vi "Principal.vi"() -> ()   [LabVIEW 2016]
uses:
  Microsoft.Kinect
  numero_imagens.vi
  <vilib>/Utility/file.llb/Write Delimited Spreadsheet (DBL).vi
  Software_TCC/historico_dados.vi
  <vilib>/University of Leeds/Kinesthesia Toolkit for Microsoft Kinect/_Polymorphic Close/Close-Skeleton and Video.vi
  <vilib>/University of Leeds/Kinesthesia Toolkit for Microsoft Kinect/_Polymorphic Configure/Event-Skeleton and Video.vi
  <vilib>/3D Express/3D Express.lvlib
panel:
  out "error out":errorcluster
  out "Status":enum16{"Default", "Aquisitar", "Calibrar Joint"}(ring)
  out "Calibraçã":bool
  in  "Cluster":T1={"Save"=FALSE, "membro"="Anatomia", "membro 2"=" Visualização", "anatomia"="Mão Esquerda", "aquisitar"=FALSE, "limpar"=FALSE, "membro"=FALSE, "calibrar_corpo"=FALSE}
  in  "Sair":bool
  in  "seleção_dados":enum32{"Capturar", "Exportar", "Config"}(tab)
  out "aceleração":dbl[](graph)
  out "velocidade":dbl[](graph)
  out "deslocamento":dbl[](graph)
  in  "kinect":string(combo)="Selecione o Kinect"
  in  "Kinect 1":string(combo)="0"
  in  "RGB":bool
  in  "membro 2":string="Status dos Kinects"
  in  "membro":string="Elevação da Câmera"
  in  "Kinect 1":bool
  out "Kinect":picture
  in  "iniciar_calibração":bool
  out "Calibrando membros":u8(slide) scale=0.0..255.0 scale format="%.6f"
  in  "Menus":enum32{"Radio Selection 4", "Radio Selection 3"}(radio)
  out "3D Picture":refnum<vi>(3d-picture)
  # "Ajustes das câmeras do Kinect"
  # "Aguarge . . ."
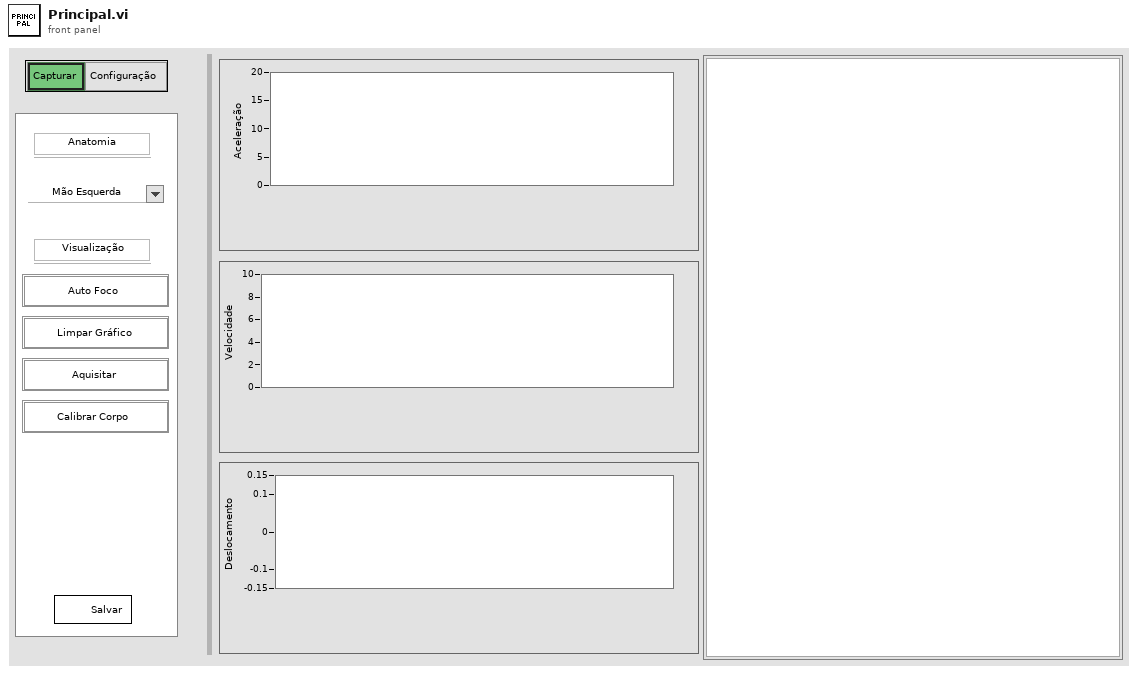
[diagram p1: front panel]
types:
  T1 = cluster{"Save":bool, "membro":string, "membro 2":string, "anatomia":string, "aquisitar":bool, "limpar":bool, "membro":bool, "calibrar_corpo":bool}
  T2 = enum8{"Enabled", "Disabled", "Disabled and Grayed Out"}
  T3 = cluster{"Scene":refnum<vi>, "Joints":refnum<vi>[], "Bones":refnum<vi>[]}
  T4 = cluster{"reference out":refnum<k24>, "KinectSensors":refnum<k24>, "SkeletonStream":refnum<k24>, "ColorStream":refnum<k24>, refnum<k24>[], "get_Item":refnum<k24>}
  T5 = cluster{cluster{"reference out":refnum<k24>, "KinectSensors":refnum<k24>}, "get_Item":refnum<k24>}
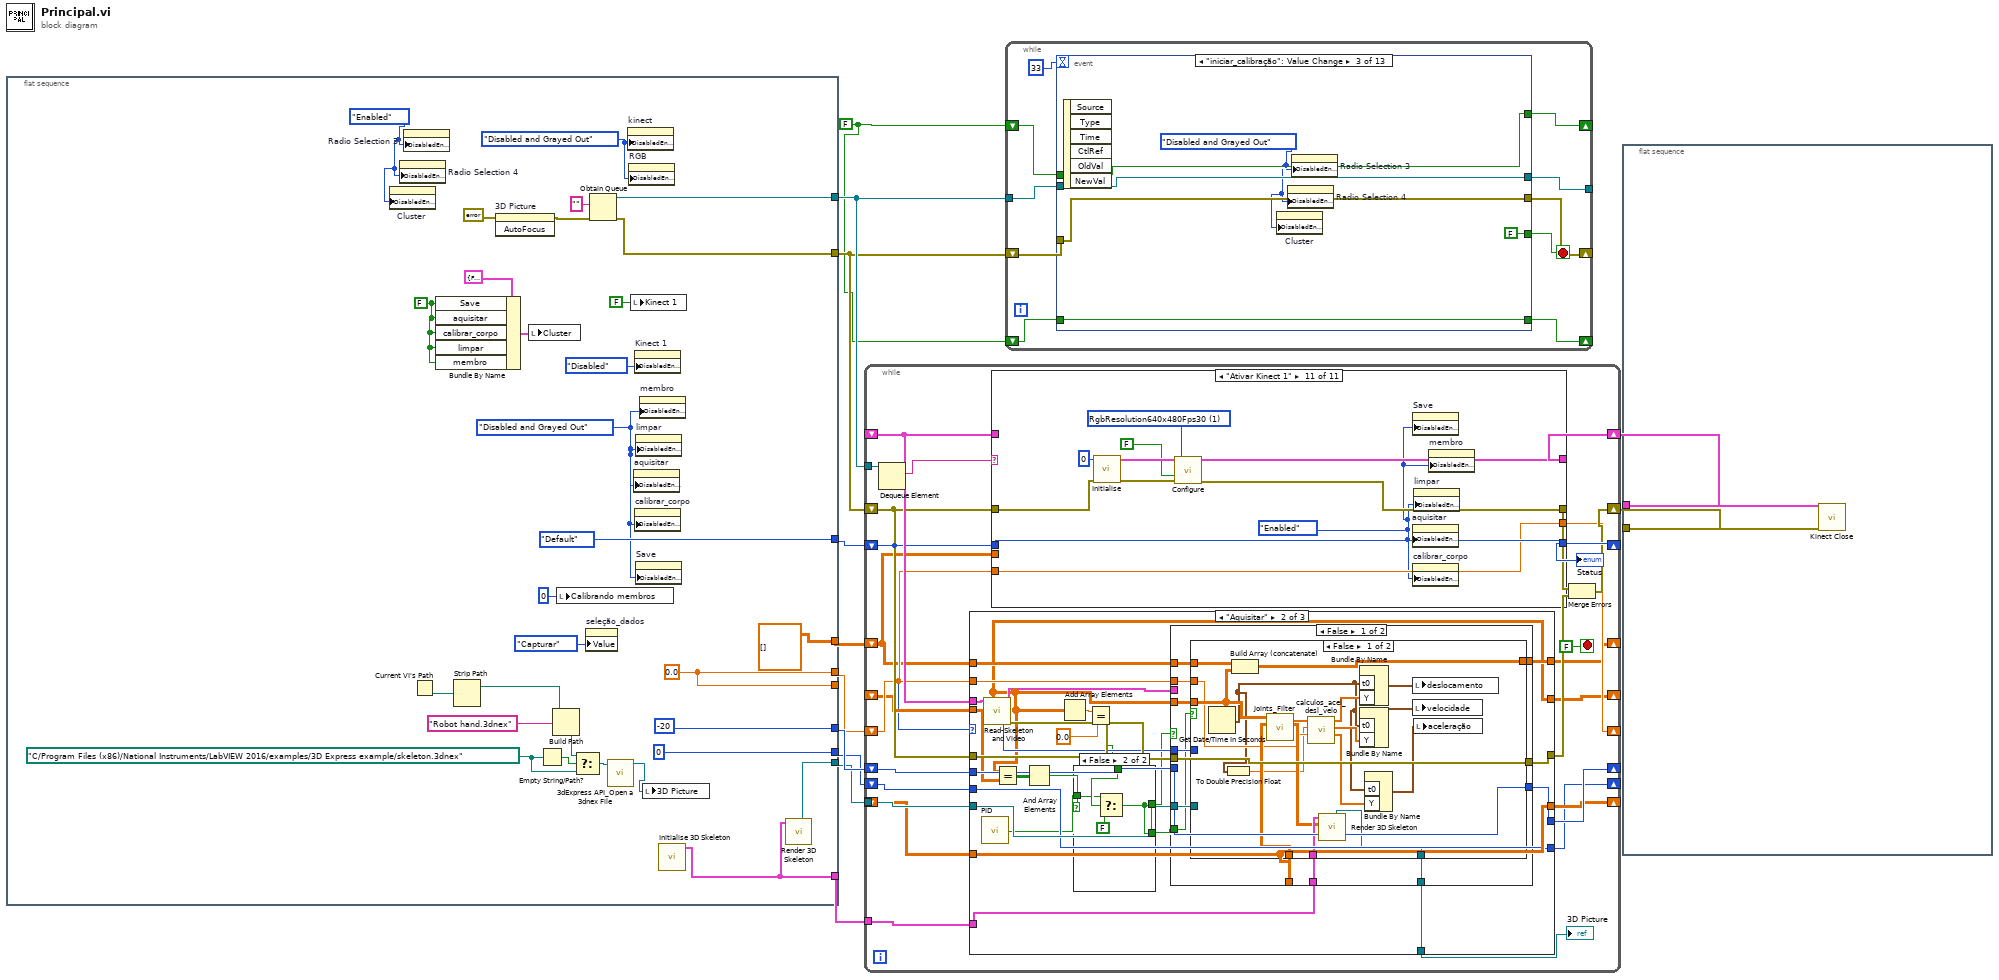
[diagram p0: block diagram]
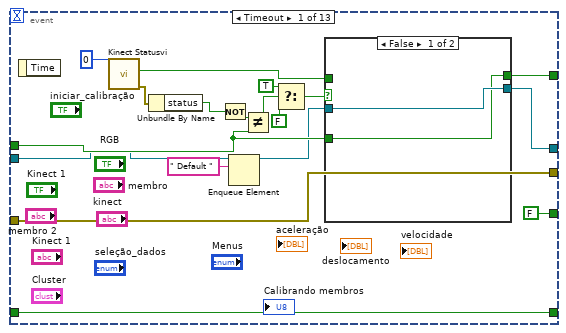
[diagram p2: hidden frame]
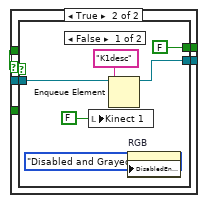
[diagram p3: hidden frame]
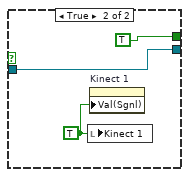
[diagram p4: hidden frame]
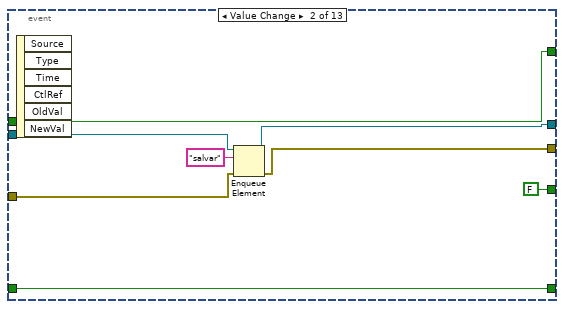
[diagram p5: hidden frame]
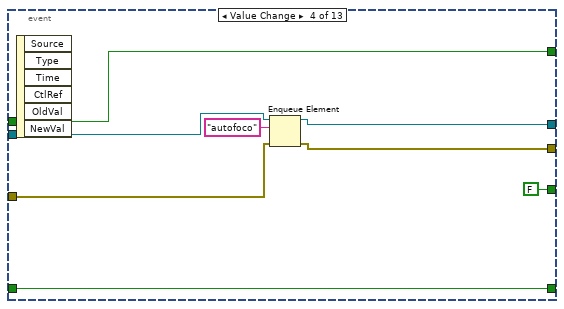
[diagram p6: hidden frame]
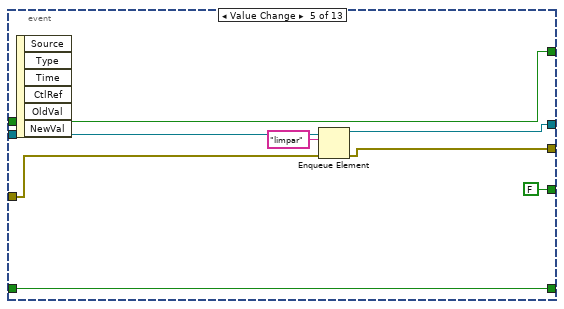
[diagram p7: hidden frame]
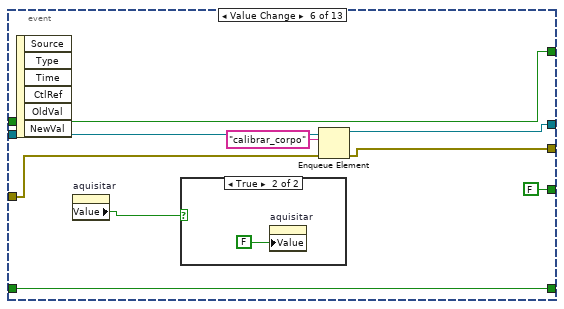
[diagram p8: hidden frame]
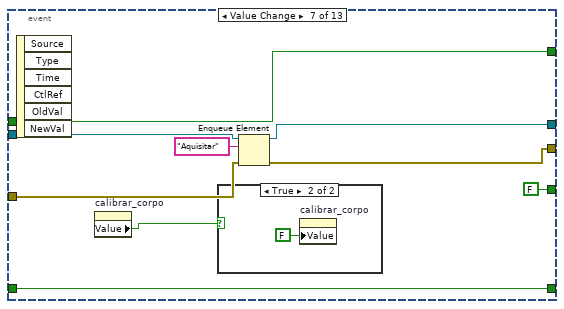
[diagram p10: hidden frame]
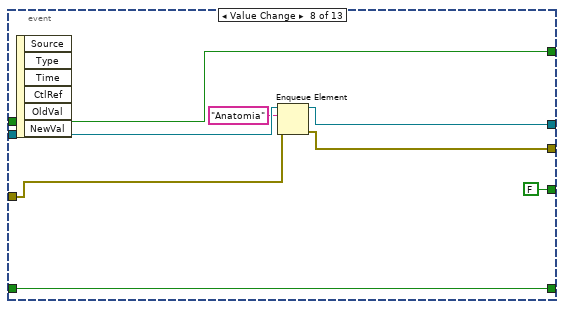
[diagram p12: hidden frame]
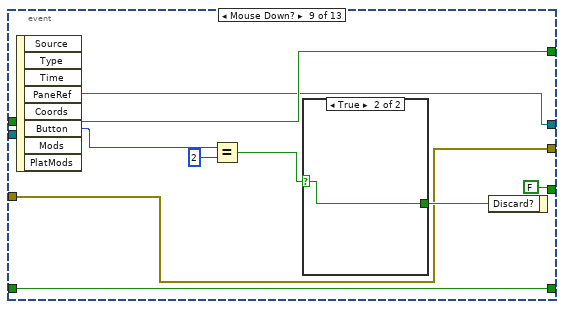
[diagram p13: hidden frame]
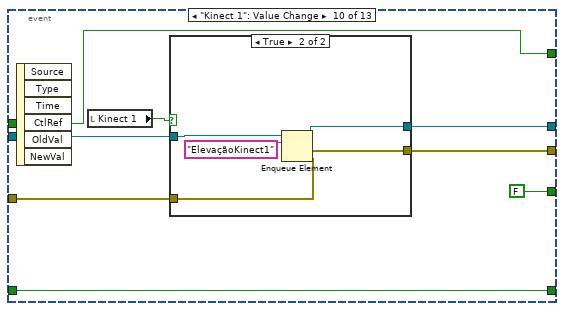
[diagram p15: hidden frame]
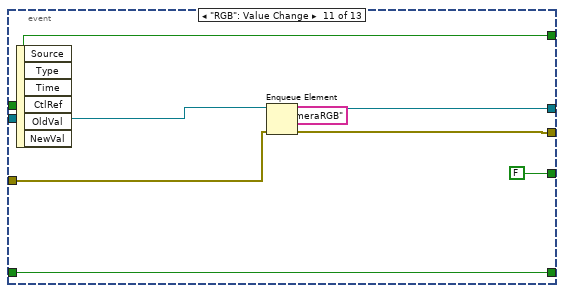
[diagram p17: hidden frame]
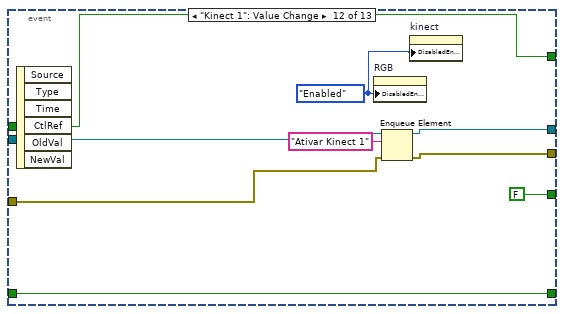
[diagram p18: hidden frame]
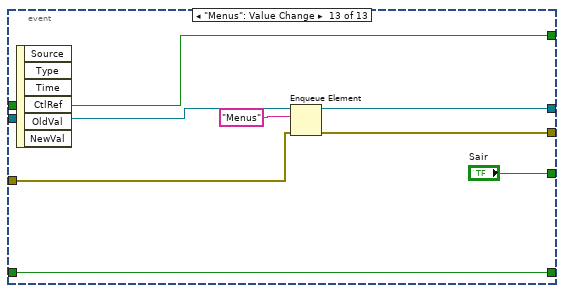
[diagram p19: hidden frame]
diagram:
  w9 = FALSE
  n1 = flat-sequence {
    tunnel: [w41] -> w12
    tunnel: [w40] -> w11
    tunnel: [enum16{"Default", "Aquisitar", "Calibrar Joint"}."Default"] -> w8
    tunnel: [-20] -> w7
    tunnel: [w26] -> w6
    tunnel: [w14] -> w4
    tunnel: [w26] -> _
    tunnel: [0] -> w3
    tunnel: [w16] -> w2
    tunnel: [dbl[][][] []] -> w1
    frame #0 {
      w13 = T2."Enabled" ("Disabled")
      w18 = FALSE ("Save")
      w23 = T2."Disabled and Grayed Out" ("Disabled")
      w28 = path "C:/Program Files (x86)/National Instruments/LabVIEW 2016/examples/3D Express example/skeleton.3dnex" ("File Path Control")
      w26 = 0.0
      w39 = T2."Disabled and Grayed Out" ("Disabled")
      n2 = property on="Cluster" class="Clust (strict)"("DisabledEnum"=w13) -> ()  [unwired: 2 in, 2 out]
      n3 = property on="Radio Selection 4" class="Bool (strict)"("DisabledEnum"=w13) -> ()  [unwired: 2 in, 2 out]
      n4 = property on="Radio Selection 3" class="Bool (strict)"("DisabledEnum"=w13) -> ()  [unwired: 2 in, 2 out]
      n5 = Current VI's Path() -> (path=w31:path)
      n6 = Bundle By Name(cluster=T1 {"Save"=FALSE, "membro"="Anatomia", "membro 2"=" Visualização", "anatomia"="Ombro Esquerdo", "aquisitar"=FALSE, "limpar"=FALSE, "membro"=FALSE, "calibrar_corpo"=FALSE} ("Cluster"), "Save"=w18, "aquisitar"=w18, "calibrar_corpo"=w18, "limpar"=w18, "membro"=w18) -> (w19:T1)
      n7 = Strip Path(path=w31) -> (stripped path=w30:path)  [unwired: 1 out]
      n8 = invoke on="3D Picture" class="SceneGraphDisp (strict)" method="AutoFocus"(error in=errorcluster {"status"=FALSE, "code"=0, "source"=""} ("error constant")) -> (error out=w35:errorcluster)  [unwired: 2 in, 2 out]
      n9 = local write "Cluster"(w19) -> ()
      n10 = Empty String/Path?(string/path=w28) -> (empty?=w29:bool)
      n11 = Build Path(base path=w30, name or relative path="Robot hand.3dnex") -> (appended path=w33:path)
      n12 = local write "Calibrando membros"(u8 0 ("Calibrando membros")) -> ()
      n13 = Select(t=w33, s=w29, f=w28) -> (s? t:f=w34:path)
      n14 = property on="seleção_dados" class="TabCtl (strict)"("Value"=enum32{"Capturar", "Exportar", "Config"}."Capturar" ("seleção_dados")) -> ()  [unwired: 2 in, 2 out]
      n15 = Obtain Queue(element data type="", error in (no error)=w35) -> (queue out=w41:refnum<queue>, error out=w40:errorcluster)  [unwired: 3 in, 1 out]
      n16 = call <vilib>:"3dExpress API_Open a 3dnex File.vi"("selected path"=w34) -> ("Scene out"=w15:refnum<vi>)  [unwired: 8 in, 2 out]
      n17 = property on="kinect" class="CmbBox"("DisabledEnum"=w39) -> ()  [unwired: 2 in, 2 out]
      n18 = property on="RGB" class="Bool"("DisabledEnum"=w39) -> ()  [unwired: 2 in, 2 out]
      n19 = local write "Kinect 1"(FALSE ("Kinect 1")) -> ()
      n20 = property on="aquisitar" class="Bool (strict)"("DisabledEnum"=w23) -> ()  [unwired: 2 in, 2 out]
      n21 = property on="Kinect 1" class="Bool (strict)"("DisabledEnum"=T2."Disabled" ("Disabled")) -> ()  [unwired: 2 in, 2 out]
      n22 = property on="calibrar_corpo" class="Bool (strict)"("DisabledEnum"=w23) -> ()  [unwired: 2 in, 2 out]
      n23 = property on="limpar" class="Bool (strict)"("DisabledEnum"=w23) -> ()  [unwired: 2 in, 2 out]
      n24 = property on="Save" class="Bool (strict)"("DisabledEnum"=w23) -> ()  [unwired: 2 in, 2 out]
      n25 = property on="membro" class="Bool (strict)"("DisabledEnum"=w23) -> ()  [unwired: 2 in, 2 out]
      n26 = local write "3D Picture"(w15) -> ()
      n27 = call <vilib>:"Initialise 3D Skeleton.vi"() -> ("Scene & Skeleton Refs"=w16:T3)  [unwired: 10 in, 1 out]
      n28 = call <vilib>:"Render 3D Skeleton.vi"("Scene & Skeleton Refs In"=w16) -> ("Scene Out"=w14:refnum<vi>)  [unwired: 7 in, 3 out]
    }
  }
  n29 = while {
    tunnel: w12 -> [w67]
    shift-right: [w57] -> w5
    shift-left: w11 -> [w62]
    shift-right: [w65] -> w10
    shift-left: _ -> [w63]
    shift-right: [w64] -> _
    shift-left: w8 -> [w43]
    shift-right: [w60] -> _
    shift-left: w7 -> [w61]
    shift-right: [w56] -> _
    shift-left: w6 -> [w55]
    tunnel: w4 -> [w54]
    shift-right: [w53] -> _
    shift-left: _ -> [w52]
    shift-right: [w51] -> _
    shift-left: _ -> [w49]
    shift-right: [w48] -> _
    shift-left: w3 -> [w50]
    tunnel: w2 -> [w46]
    shift-right: [w45] -> _
    shift-left: w1 -> [w44]
    stop <- FALSE stop-if-true
    n30 = Dequeue Element(queue=w67) -> (element=w66:string)  [unwired: 2 in, 3 out]
    n31 = case shown="\"Aquisitar\"" w43 {
      tunnel: w63 -> [_ w101 w183]
      tunnel: w62 -> [w75 w100 w182]
      tunnel: [w75 w91 w171] -> w59
      tunnel: w61 -> [w74 w94 w176]
      tunnel: [w74 w93 w175] -> w60
      tunnel: w55 -> [_ w92 w174]
      tunnel: w54 -> [w70 w90 w170]
      tunnel: [w73 w77 w157] -> w53
      tunnel: w52 -> [w73 w89 w169]
      tunnel: [w72 w87 w166] -> w51
      tunnel: w50 -> [w71 w86 w167]
      tunnel: w49 -> [w72 w87 w165]
      tunnel: [w71 w86 w162] -> w48
      tunnel: [w70 w85 w159] -> w47
      tunnel: w46 -> [_ w76 w160]
      tunnel: w44 -> [w69 w79 w156]
      tunnel: [w69 w78 w156] -> w45
      frame "Default", Default {
      }
      frame "Aquisitar" {
        n32 = call "PID"() -> ("Time has Elapsed"=w81:bool)  [unwired: 12 in, 7 out]
        n33 = call <vilib>:"Read-Skeleton and Video.vi"("Kinect References in"=w101, "error in (no error)"=w100) -> ("Primary Skeleton Array"=w77:dbl[][], "Kinect References out"=w95:T4, "Timestamp"=w98:u32, "error out"=w99:errorcluster)  [unwired: 9 in, 1 out]
        n34 = Equal?(x=w77, y=w89) -> (x = y?=w88:bool[][])
        n35 = And Array Elements(Boolean array=w88) -> (logical AND=w80:bool)
        n36 = Add Array Elements(numeric array=w77) -> (sum=w97:dbl)
        n37 = Equal?(x=w97, y=0.0) -> (x = y?=w84:bool)
        n38 = case shown="False" w80 {
          tunnel: [w103 w111] -> w82
          tunnel: w84 -> [w107 w110]
          tunnel: [w104 w111] -> w83
          tunnel: w81 -> [w102 w109]
          frame True {
            n39 = Select(t=TRUE ("f"), s=w107, f=FALSE) -> (s? t:f=w104:bool)
            n40 = Select(t=w102, s=w107, f=FALSE) -> (s? t:f=w103:bool)
          }
          frame False {
            n41 = Select(t=w109, s=w110, f=FALSE) -> (s? t:f=w111:bool)
          }
        }
        n42 = case shown="False" w82 {
          tunnel: w99 -> [w122 _]
          tunnel: [w122 w147] -> w91
          tunnel: w77 -> [w124 _]
          tunnel: w98 -> [w123 _]
          tunnel: w95 -> [_ w154]
          tunnel: w94 -> [w121 w150]
          tunnel: [w121 w146] -> w93
          tunnel: w92 -> [w120 _]
          tunnel: w90 -> [w119 w145]
          tunnel: w87 -> [w118 _]
          tunnel: [w117 w145] -> w85
          tunnel: w83 -> [w116 _]
          tunnel: w79 -> [w115 w144]
          tunnel: [w114 w144] -> w78
          tunnel: w76 -> [w113 _]
          frame False {
            n43 = case shown="False" w116 {
              tunnel: w124 -> [w134 _]
              tunnel: w123 -> [_ _]
              tunnel: w120 -> [w127 _]
              tunnel: w119 -> [_ w143]
              tunnel: w118 -> [w129 _]
              tunnel: [w131 w143] -> w117
              tunnel: w115 -> [w133 w142]
              tunnel: [w132 w142] -> w114
              tunnel: w113 -> [w130 _]
              frame False {
                n44 = Get Date/Time In Seconds() -> (seconds since 1Jan1904=w126:timestamp)
                n45 = To Double Precision Float(number=w126) -> (double precision float=w125:dbl)
                n46 = Build Array (concatenate)(w133, w134) -> (w132:dbl[][][])
                n47 = call "Joints_Filter.vi"("Modelo"=w129, "Kinect 1"=w134) -> ("Array Válido"=w128:dbl[][], "Joints"=w135:dbl[])  [unwired: 8 in]
                n48 = call "calculos_acel_desl_velo.vi"("Numeric Control"=w127, "TimeStamp"=w125, "Joints"=w135) -> ("Aceleração"=w139:dbl[], "Velocidade"=w138:dbl[], "Deslocamento"=w141:dbl[])  [unwired: 6 in]
                n49 = call <vilib>:"Render 3D Skeleton.vi"("Array of Joint Positions"=w128, "Scene & Skeleton Refs In"=w130) -> ("Scene Out"=w131:refnum<vi>)  [unwired: 6 in, 3 out]
                n50 = Bundle By Name("t0"=w126, "Y"=w141) -> (w140:waveform(dbl))  [unwired: 1 in]
                n51 = Bundle By Name("t0"=w126, "Y"=w138) -> (w136:waveform(dbl))  [unwired: 1 in]
                n52 = Bundle By Name("t0"=w126, "Y"=w139) -> (w137:waveform(dbl))  [unwired: 1 in]
                n53 = local write "deslocamento"(w140) -> ()
                n54 = local write "velocidade"(w136) -> ()
                n55 = local write "aceleração"(w137) -> ()
              }
              frame True {
              }
            }
          }
          frame True {
            n56 = Unbundle By Name(w154) -> ("get_Item"=w155:refnum<k24>)
            n57 = Greater?(x=w150, y=20) -> (0:w152:bool)
            n58 = Add(x=w150, y=10) -> (x+y=w148:i32)
            n59 = Select(t=-20 ("y"), s=w152, f=w148) -> (s? t:f=w146:i32)
            n60 = property class="KinectSensor"(reference=w155, "ElevationAngle"=w146) -> (error out=w147:errorcluster)  [unwired: 1 in, 1 out]
          }
        }
      }
      frame "Calibrar Joint" {
        n61 = call "PID2"() -> ("Time has Elapsed"=w173:bool)  [unwired: 12 in, 7 out]
        n62 = call <vilib>:"Read-Skeleton and Video.vi"("Kinect References in"=w183, "error in (no error)"=w182) -> ("Primary Skeleton Array"=w157:dbl[][], "Kinect References out"=w177:T4, "Timestamp"=w180:u32, "error out"=w181:errorcluster)  [unwired: 9 in, 1 out]
        n63 = Equal?(x=w157, y=w169) -> (x = y?=w168:bool[][])
        n64 = local read "iniciar_calibração"() -> (w158:bool)
        n65 = And Array Elements(Boolean array=w168) -> (logical AND=w163:bool)
        n66 = Add Array Elements(numeric array=w157) -> (sum=w179:dbl)
        n67 = call <vilib>:"Render 3D Skeleton.vi"("Array of Joint Positions"=w157, "Scene & Skeleton Refs In"=w160) -> ("Scene Out"=w159:refnum<vi>)  [unwired: 6 in, 3 out]
        n68 = Equal?(x=w179, y=0.0) -> (x = y?=w164:bool)
        n69 = case shown="True" w163 {
          tunnel: w173 -> [w190 w194]
          tunnel: [w184 w191] -> w172
          tunnel: w164 -> [w188 w192]
          tunnel: [w185 w191] -> w161
          frame True {
            n70 = Select(t=TRUE ("f"), s=w188, f=FALSE) -> (s? t:f=w185:bool)
            n71 = Select(t=w190, s=w188, f=FALSE) -> (s? t:f=w184:bool)
          }
          frame False {
            n72 = Select(t=w194, s=w192, f=FALSE) -> (s? t:f=w191:bool)
          }
        }
        n73 = case shown="False" w172 {
          tunnel: w181 -> [w204 _]
          tunnel: [w204 w238] -> w171
          tunnel: w157 -> [w206 _]
          tunnel: w180 -> [w205 _]
          tunnel: w177 -> [_ w245]
          tunnel: w176 -> [w203 w241]
          tunnel: [w203 w237] -> w175
          tunnel: w174 -> [w202 _]
          tunnel: w170 -> [w198 w235]
          tunnel: w167 -> [w201 w234]
          tunnel: [w200 w236] -> w166
          tunnel: w165 -> [w199 w236]
          tunnel: [w198 w235] -> _
          tunnel: [w197 w234] -> w162
          tunnel: w161 -> [w196 _]
          tunnel: w158 -> [w195 _]
          frame False {
            n74 = case shown="True" w196 {
              tunnel: w206 -> [w214 _]
              tunnel: w205 -> [w213 _]
              tunnel: w202 -> [w212 _]
              tunnel: w201 -> [w211 w232]
              tunnel: [w210 w233] -> w200
              tunnel: w199 -> [w209 w233]
              tunnel: [w208 w232] -> w197
              tunnel: w195 -> [w207 _]
              frame False {
                n75 = case shown="True" w207 {
                  tunnel: w214 -> [_ w220]
                  tunnel: w213 -> [_ _]
                  tunnel: w212 -> [_ _]
                  tunnel: w211 -> [w215 w227]
                  tunnel: [w216 w224] -> w210
                  tunnel: w209 -> [w216 w223]
                  tunnel: [w215 w222] -> w208
                  frame False {
                  }
                  frame True {
                    n76 = call "cal_joints padrao.vi"("Joints"=w220) -> ()  [unwired: 11 in]
                    n77 = Increment(x=w227) -> (x+1=w217:i32)
                    n78 = global write "numero_imagens.vi" "Número de Imagens"(w217) -> ()
                    n79 = global read "historico_calibraçcao.vi" "Histórico"() -> (w219:dbl[][])
                    n80 = Divide(x=w217, y=6.66) -> (x/y=w218:dbl)
                    n81 = Greater?(x=w217, y=1700) -> (0:w225:bool)
                    "Calibraçã" <- w225
                    n82 = local write "Calibrando membros"(w218) -> ()
                    n83 = case shown="True" w225 {
                      tunnel: w219 -> [_ w230]
                      tunnel: [w229 w230] -> w224
                      tunnel: w223 -> [w229 _]
                      tunnel: [w228 0] -> w222
                      tunnel: w217 -> [w228 _]
                      frame False {
                      }
                      frame True {
                      }
                    }
                  }
                }
              }
              frame True {
              }
            }
          }
          frame True {
            n84 = Unbundle By Name(w245) -> ("get_Item"=w246:refnum<k24>)
            n85 = Greater?(x=w241, y=20) -> (0:w243:bool)
            n86 = Add(x=w241, y=10) -> (x+y=w239:i32)
            n87 = Select(t=-20 ("y"), s=w243, f=w239) -> (s? t:f=w237:i32)
            n88 = property class="KinectSensor"(reference=w246, "ElevationAngle"=w237) -> (error out=w238:errorcluster)  [unwired: 1 in, 1 out]
          }
        }
      }
    }
    "3D Picture" <- w47
    n89 = case shown="\"Ativar Kinect 1\"" w66 {
      tunnel: w62 -> [w251 w274 w302 w305 w314 w325 w335 w345 w361 w372 w383]
      tunnel: [w252 w273 w299 w306 w317 w326 w338 w347 w363 T4 {"reference out"=refnum, "KinectSensors"=refnum, "SkeletonStream"=refnum, "ColorStream"=refnum, [], "get_Item"=refnum} ("Kinect References out") w378] -> w65
      tunnel: [w251 w264 w296 w305 w314 w325 w335 w346 w364 w369 w377] -> w58
      tunnel: w63 -> [w252 w273 w299 w306 w317 w326 w338 w348 w363 w373 _]
      tunnel: [w248 w276 w300 w304 w315 w327 w337 w343 w358 enum16{"Default", "Aquisitar", "Calibrar Joint"}."Default" w376] -> w64
      tunnel: w43 -> [w247 w276 w300 w304 _ _ w337 w343 w358 _ w376]
      tunnel: [w250 w275 w301 w303 w318 w324 w336 w342 w357 w367 w375] -> w56
      tunnel: w55 -> [w250 w275 w301 w303 w318 w324 _ w342 w357 w367 w375]
      tunnel: w44 -> [_ w277 _ _ _ _ _ _ _ _ _]
      frame Default {
        n90 = local read "Calibraçã"() -> (w249:bool)
        n91 = case shown="True" w249 {
          tunnel: [w253 enum16{"Default", "Aquisitar", "Calibrar Joint"}."Default"] -> w248
          tunnel: w247 -> [w254 _]
          frame False {
            w256 = enum16{"Default", "Aquisitar", "Calibrar Joint"}."Calibrar Joint" ("y")
            n92 = Equal?(x=w254, y=w256) -> (x = y?=w255:bool)
            n93 = property on="aquisitar" class="Bool (strict)" props=["Value"]() -> ()  [unwired: 2 in, 3 out]
            n94 = Select(t=w256, s=w255, f=w254) -> (s? t:f=w253:enum16{"Default", "Aquisitar", "Calibrar Joint"})
          }
          frame True {
            w257 = T2."Enabled" ("Disabled")
            w259 = FALSE ("Calibraçã")
            n95 = local write "Calibrando membros"(u8 0 ("Calibrando membros")) -> ()
            n96 = property on="seleção_dados" class="TabCtl (strict)"("Value"=enum32{"Capturar", "Exportar", "Config"}."Capturar" ("seleção_dados")) -> ()  [unwired: 2 in, 2 out]
            n97 = global write "historico_calibraçcao.vi" "Histórico"(dbl[][] [] ("Histórico")) -> ()
            n98 = local write "Calibraçã"(w259) -> ()
            n99 = property on="calibrar_corpo" class="Bool (strict)"("Value"=w259) -> ()  [unwired: 2 in, 2 out]
            n100 = property on="iniciar_calibração" class="Bool (strict)"("Value"=w259) -> ()  [unwired: 2 in, 2 out]
            n101 = One Button Dialog(message="Calibração terminada com Sucesso!.") -> ()  [unwired: 1 in, 1 out]
            n102 = property on="Radio Selection 4" class="Bool (strict)"("DisabledEnum"=w257) -> ()  [unwired: 2 in, 2 out]
            n103 = property on="Radio Selection 3" class="Bool (strict)"("DisabledEnum"=w257) -> ()  [unwired: 2 in, 2 out]
            n104 = property on="Cluster" class="Clust (strict)"("DisabledEnum"=w257) -> ()  [unwired: 2 in, 2 out]
          }
        }
      }
      frame "salvar" {
        n105 = call "File Dialog"() -> ("selected path"=w271:path, "error out"=w267:errorcluster)  [unwired: 12 in, 2 out]
        n106 = call <vilib>:"Check if File or Folder Exists.vi"("path"=w271) -> ("file or folder exists?"=w270:bool, "dup path"=w269:path)  [unwired: 8 in, 1 out]
        n107 = case shown="True" w270 {
          tunnel: w269 -> [w282 w284]
          tunnel: [w281 w284] -> w268
          tunnel: [w280 w283] -> w266
          tunnel: w267 -> [_ w283]
          frame False {
            n108 = Create Folder(path (use dialog)=w282) -> (created path=w281:path, error out=w280:errorcluster)  [unwired: 2 in, 1 out]
          }
          frame True {
          }
        }
        "error out" <- w266
        n109 = for {
          tunnel: w277 -> [w292] mode=indexing
          tunnel: [w290] -> w265
          tunnel: w274 -> [w289]
          tunnel: w268 -> [w285]
          i -> [w295]
          n110 = Increment(x=w295) -> (x+1=w294:i32)
          n111 = Number To Decimal String(number=w294) -> (decimal integer string=w288:string)  [unwired: 1 in]
          n112 = Concatenate Strings(w288, ".csv" ("string")) -> (w287:string)
          n113 = Build Path(base path=w285, name or relative path=w287) -> (appended path=w293:path)
          n114 = call-poly <vilib>:"Write Delimited Spreadsheet.vi"("file path (dialog if empty)"=w293, "2D data"=w292, "error in (no error)"=w289, "delimiter (\\t)"=";" ("delimiter (\\t)")) -> ("error out"=w290:errorcluster)  [unwired: 10 in, 1 out]
        }
        n115 = flat-sequence {
          tunnel: [w278] -> w264
          tunnel: w265 -> [w278]
          frame #0 {
            n116 = One Button Dialog(message="Salvo com sucesso.") -> ()  [unwired: 1 in, 1 out]
          }
        }
        n117 = property on="Save" class="Bool (strict)"("Value"=FALSE) -> ()  [unwired: 2 in, 2 out]
      }
      frame "autofoco" {
        n118 = invoke on="3D Picture" class="SceneGraphDisp (strict)" method="AutoFocus"(error in=w302) -> (error out=w297:errorcluster)  [unwired: 2 in, 2 out]
        n119 = property on="membro" class="Bool (strict)"(error in=w297, "Value"=FALSE ("Value (Signaling)")) -> (error out=w296:errorcluster)  [unwired: 1 in, 1 out]
      }
      frame "Menus" {
        n120 = local read "Menus"() -> (w307:enum32{"Radio Selection 4", "Radio Selection 3"})
        n121 = case shown="\"Radio Selection 4\", Default" w307 {
          frame "Radio Selection 4", Default {
            n122 = property on="Cluster" class="Clust (strict)"("DisabledEnum"=T2."Enabled" ("Disabled")) -> ()  [unwired: 2 in, 2 out]
            n123 = property on="seleção_dados" class="TabCtl (strict)"("Value"=enum32{"Capturar", "Exportar", "Config"}."Capturar" ("seleção_dados")) -> ()  [unwired: 2 in, 2 out]
            n124 = property on="seleção_dados" class="TabCtl (strict)"("Value"=enum32{"Capturar", "Exportar", "Config"}."Capturar" ("seleção_dados")) -> ()  [unwired: 2 in, 2 out]
          }
          frame "Radio Selection 3" {
            n125 = property on="Cluster" class="Clust (strict)"("DisabledEnum"=T2."Disabled and Grayed Out" ("Disabled")) -> ()  [unwired: 2 in, 2 out]
            n126 = property on="seleção_dados" class="TabCtl (strict)"("Value"=enum32{"Capturar", "Exportar", "Config"}."Exportar" ("seleção_dados")) -> ()  [unwired: 2 in, 2 out]
            n127 = property on="seleção_dados" class="TabCtl (strict)"("Value"=enum32{"Capturar", "Exportar", "Config"}."Exportar" ("seleção_dados")) -> ()  [unwired: 2 in, 2 out]
          }
        }
      }
      frame "calibrar_corpo" {
        n128 = property on="calibrar_corpo" class="Bool (strict)"() -> ("Value"=w316:bool)  [unwired: 2 in, 2 out]
        n129 = case shown="True" w316 {
          tunnel: [enum16{"Default", "Aquisitar", "Calibrar Joint"}."Default" enum16{"Default", "Aquisitar", "Calibrar Joint"}."Calibrar Joint"] -> w315
          frame False {
            n130 = global write "numero_imagens.vi" "Número de Imagens"(0.0 ("Número de Imagens")) -> ()
            n131 = property on="seleção_dados" class="TabCtl (strict)"("Value"=enum32{"Capturar", "Exportar", "Config"}."Capturar" ("seleção_dados")) -> ()  [unwired: 2 in, 2 out]
          }
          frame True {
            n132 = property on="seleção_dados" class="TabCtl (strict)"("Value"=enum32{"Capturar", "Exportar", "Config"}."Config" ("seleção_dados")) -> ()  [unwired: 2 in, 2 out]
          }
        }
      }
      frame "Aquisitar" {
        n133 = local read "Cluster"() -> (w329:T1)
        n134 = Unbundle By Name(w329) -> ("aquisitar"=w328:bool)
        n135 = case shown="True" w328 {
          tunnel: [enum16{"Default", "Aquisitar", "Calibrar Joint"}."Default" enum16{"Default", "Aquisitar", "Calibrar Joint"}."Aquisitar"] -> w327
          frame False {
          }
          frame True {
            n136 = property on="seleção_dados" class="TabCtl (strict)"("Value"=enum32{"Capturar", "Exportar", "Config"}."Capturar" ("seleção_dados")) -> ()  [unwired: 2 in, 2 out]
          }
        }
      }
      frame "Anatomia" {
        w334 = dbl[] [] ("deslocamento")
        n137 = local read "Cluster"() -> (w341:T1)
        n138 = Unbundle By Name(w341) -> ("anatomia"=w339:string)
        n139 = property on="anatomia" class="CmbBox"() -> ("Strings[]"=w340:string[])  [unwired: 2 in, 2 out]
        n140 = Search 1D Array(1D array=w340, element=w339) -> (index of element=w336:i32)  [unwired: 1 in]
        n141 = global write "historico_dados.vi" "Histórico"(dbl[][] [] ("Histórico")) -> ()
        n142 = local write "deslocamento"(w334) -> ()
        n143 = local write "velocidade"(w334) -> ()
        n144 = local write "aceleração"(w334) -> ()
      }
      frame "CameraRGB" {
        n145 = property on="kinect" class="CmbBox"() -> ("Value"=w344:string)  [unwired: 2 in, 2 out]
        n146 = case shown="\"False\", Default" w344 {
          tunnel: w348 -> [w350 w355]
          tunnel: [w350 w353] -> w347
          tunnel: [w349 w352] -> w346
          tunnel: w345 -> [w349 w351]
          frame "False", Default {
          }
          frame "Kinect 1" {
            n147 = call-poly <vilib>:"Read.vi"("Kinect References in"=w355, "error in (no error)"=w351) -> ("Colour output array (U24, RGB)"=w354:u32[][], "Kinect References out"=w353:T4, "error out"=w352:errorcluster)  [unwired: 9 in, 2 out]
            n148 = call <vilib>:"Display Colour Data (U32 to picture).vi"("Colour output array (U24, RGB)"=w354) -> ("new picture"=→"Kinect":picture)  [unwired: 10 in]
          }
        }
      }
      frame "ElevaçãoKinect1" {
        n149 = Unbundle By Name(w363) -> ("get_Item"=w365:refnum<k24>)
        n150 = property on="Kinect 1" class="CmbBox"(error in=w361) -> (error out=w359:errorcluster, "Value"=w360:string)  [unwired: 1 in, 1 out]
        n151 = Decimal String To Number(string=w360) -> (number=w362:i32)  [unwired: 2 in, 1 out]
        n152 = property class="KinectSensor"(reference=w365, error in=w359, "ElevationAngle"=w362) -> (error out=w364:errorcluster)  [unwired: 1 out]
      }
      frame "K1desc" {
        w366 = T2."Disabled and Grayed Out" ("Disabled")
        n153 = call-poly <vilib>:"Kinect Close.vi"("Kinect References in"=w373, "error in"=w372) -> ("error out"=w370:errorcluster)  [unwired: 13 in]
        n154 = call <vilib>:"Clear Errors.vi"("error in (no error)"=w370) -> ("error out"=w369:errorcluster)  [unwired: 5 in, 1 out]
        n155 = property on="Save" class="Bool (strict)"("DisabledEnum"=w366) -> ()  [unwired: 2 in, 2 out]
        n156 = property on="aquisitar" class="Bool (strict)"("DisabledEnum"=w366) -> ()  [unwired: 2 in, 2 out]
        n157 = property on="calibrar_corpo" class="Bool (strict)"("DisabledEnum"=w366) -> ()  [unwired: 2 in, 2 out]
        n158 = property on="limpar" class="Bool (strict)"("DisabledEnum"=w366) -> ()  [unwired: 2 in, 2 out]
        n159 = property on="membro" class="Bool (strict)"("DisabledEnum"=w366) -> ()  [unwired: 2 in, 2 out]
      }
      frame "Ativar Kinect 1" {
        w374 = T2."Enabled" ("Disabled")
        w380 = 1 items=["Undefined", "RgbResolution640x480Fps30", "RgbResolution1280x960Fps12", "YuvResolution640x480Fps15", "RawYuvResolution640x480Fps15"] ("RGB Stream Format")
        n160 = call <vilib>:"Initialise.vi"("Kinect Number"=0, "error in (no error)"=w383) -> ("Kinect References out"=w382:T5, "error out"=w381:errorcluster)  [unwired: 12 in]
        n161 = call-poly <vilib>:"Configure.vi"("Kinect References in"=w382, "RGB Stream Format"=w380, "Skeleton Smoothing"=FALSE, "error in"=w381) -> ("Kinect References out"=w378:T4, "error out"=w377:errorcluster)  [unwired: 10 in]
        n162 = property on="aquisitar" class="Bool (strict)"("DisabledEnum"=w374) -> ()  [unwired: 2 in, 2 out]
        n163 = property on="Save" class="Bool (strict)"("DisabledEnum"=w374) -> ()  [unwired: 2 in, 2 out]
        n164 = property on="calibrar_corpo" class="Bool (strict)"("DisabledEnum"=w374) -> ()  [unwired: 2 in, 2 out]
        n165 = property on="limpar" class="Bool (strict)"("DisabledEnum"=w374) -> ()  [unwired: 2 in, 2 out]
        n166 = property on="membro" class="Bool (strict)"("DisabledEnum"=w374) -> ()  [unwired: 2 in, 2 out]
      }
    }
    "Status" <- w64
    n167 = Merge Errors(w58, w59) -> (w57:errorcluster)
  }
  n168 = while {
    tunnel: w12 -> [w392]
    shift-right: [w390] -> _
    shift-left: w11 -> [w393]
    tunnel: [w391] -> _
    shift-right: [w387] -> _
    shift-left: w9 -> [w388]
    shift-right: [w385] -> _
    shift-left: w9 -> [w386]
    stop <- w394 stop-if-true
    n169 = event shown="[2] \"iniciar_calibração\": Value Change" {
      selector: _ -> [_ _ _ _ _ _ _ _ _ _ _ _ _]
      dyn-events: _ -> [_ _ _ _ _ _ _ _ _ _ _ _ _]
      timeout: 33 -> [_ _ _ _ _ _ _ _ _ _ _ _ _]
      tunnel: [FALSE FALSE ("Sair") FALSE ("Sair") FALSE ("Sair") FALSE ("Sair") FALSE ("Sair") FALSE ("Sair") FALSE ("Sair") FALSE ("Sair") FALSE ("Sair") FALSE ("Sair") FALSE ("Sair") "Sair"] -> w394
      tunnel: w393 -> [w411 w434 w439 w445 w454 w463 w473 w479 w487 w501 w516 w526 w536]
      tunnel: w392 -> [w397 w435 w441 w448 w457 w466 w476 w485 w488 w503 w519 w528 w535]
      tunnel: [w408 w428 w441 w446 w456 w465 w475 w483 w488 w502 w518 w527 w534] -> w391
      tunnel: [w411 w433 w439 w444 w453 w462 w474 w478 w487 w500 w517 w525 w533] -> w390
      tunnel: w388 -> [w405 w431 w440 w442 w455 w464 w471 w482 w489 w498 w513 w523 w530]
      tunnel: [w407 w431 w440 w442 w455 w464 w471 w482 w489 w498 w513 w523 w530] -> w387
      tunnel: w386 -> [w398 w430 w437 w447 w451 w460 w469 w481 w486 w497 w512 w520 w529]
      tunnel: [w398 w430 w437 w447 w451 w460 w469 w481 w486 w497 w512 w520 w529] -> w385
      event Timeout {
        n170 = event-data() -> ()  [unwired: 1 in, 1 out]
        n171 = call "Kinect Statusvi.vi"("Kinect"=0) -> ("error out"=w399:errorcluster, "Conectado"=w406:bool)  [unwired: 8 in, 1 out]
        n172 = Unbundle By Name(w399) -> ("status"=w401:bool)
        n173 = Not(x=w401) -> (.not. x?=w400:bool)
        n174 = Enqueue Element(queue=w397, element=" Default ") -> (queue out=w396:refnum<queue>)  [unwired: 2 in, 2 out]
        n175 = Not Equal?(x=w400, y=w405) -> (x != y?=w404:bool)
        n176 = Select(t=TRUE, s=w404, f=FALSE) -> (s? t:f=w410:bool)
        n177 = case shown="False" w410 {
          tunnel: w396 -> [w414 w418]
          tunnel: [w414 w417] -> w408
          tunnel: [w413 w416] -> w407
          tunnel: w405 -> [w413 _]
          tunnel: w406 -> [_ w415]
          frame False {
          }
          frame True {
            n178 = case shown="False" w415 {
              tunnel: w418 -> [w424 w427]
              tunnel: [w423 w427] -> w417
              tunnel: [FALSE TRUE] -> w416
              frame False {
                n179 = local write "Kinect 1"(FALSE ("Kinect 1")) -> ()
                n180 = Enqueue Element(queue=w424, element="K1desc") -> (queue out=w423:refnum<queue>)  [unwired: 2 in, 2 out]
                n181 = property on="RGB" class="Bool"("DisabledEnum"=T2."Disabled and Grayed Out" ("Disabled")) -> ()  [unwired: 2 in, 2 out]
              }
              frame True {
                w426 = TRUE ("Kinect 1")
                n182 = local write "Kinect 1"(w426) -> ()
                n183 = property on="Kinect 1" class="Bool (strict)"("Val(Sgnl)"=w426) -> ()  [unwired: 2 in, 2 out]
              }
            }
          }
        }
      }
      event "Cluster.Save": Value Change {
        n184 = event-data() -> ()  [unwired: 1 in, 6 out]
        n185 = Enqueue Element(queue=w435, element="salvar", error in (no error)=w434) -> (queue out=w428:refnum<queue>, error out=w433:errorcluster)  [unwired: 1 in, 1 out]
      }
      event "iniciar_calibração": Value Change {
        w436 = T2."Disabled and Grayed Out" ("Disabled")
        n186 = event-data() -> ()  [unwired: 1 in, 6 out]
        n187 = property on="Cluster" class="Clust (strict)"("DisabledEnum"=w436) -> ()  [unwired: 2 in, 2 out]
        n188 = property on="Radio Selection 4" class="Bool (strict)"("DisabledEnum"=w436) -> ()  [unwired: 2 in, 2 out]
        n189 = property on="Radio Selection 3" class="Bool (strict)"("DisabledEnum"=w436) -> ()  [unwired: 2 in, 2 out]
      }
      event "Cluster.membro": Value Change {
        n190 = event-data() -> ()  [unwired: 1 in, 6 out]
        n191 = Enqueue Element(queue=w448, element="autofoco", error in (no error)=w445) -> (queue out=w446:refnum<queue>, error out=w444:errorcluster)  [unwired: 1 in, 1 out]
      }
      event "Cluster.limpar": Value Change {
        n192 = event-data() -> ()  [unwired: 1 in, 6 out]
        n193 = Enqueue Element(queue=w457, element="limpar", error in (no error)=w454) -> (queue out=w456:refnum<queue>, error out=w453:errorcluster)  [unwired: 1 in, 1 out]
      }
      event "Cluster.calibrar_corpo": Value Change {
        n194 = event-data() -> ()  [unwired: 1 in, 6 out]
        n195 = property on="aquisitar" class="Bool (strict)"() -> ("Value"=w458:bool)  [unwired: 2 in, 2 out]
        n196 = case shown="True" w458 {
          frame False {
          }
          frame True {
            n197 = property on="aquisitar" class="Bool (strict)"("Value"=FALSE ("Value (Signaling)")) -> ()  [unwired: 2 in, 2 out]
          }
        }
        n198 = Enqueue Element(queue=w466, element="calibrar_corpo", error in (no error)=w463) -> (queue out=w465:refnum<queue>, error out=w462:errorcluster)  [unwired: 1 in, 1 out]
      }
      event "Cluster.aquisitar": Value Change {
        n199 = event-data() -> ()  [unwired: 1 in, 6 out]
        n200 = property on="calibrar_corpo" class="Bool (strict)"() -> ("Value"=w468:bool)  [unwired: 2 in, 2 out]
        n201 = case shown="True" w468 {
          frame False {
          }
          frame True {
            n202 = property on="calibrar_corpo" class="Bool (strict)"("Value"=FALSE) -> ()  [unwired: 2 in, 2 out]
          }
        }
        n203 = Enqueue Element(queue=w476, element="Aquisitar", error in (no error)=w473) -> (queue out=w475:refnum<queue>, error out=w474:errorcluster)  [unwired: 1 in, 1 out]
      }
      event "Cluster.anatomia": Value Change {
        n204 = event-data() -> ()  [unwired: 1 in, 6 out]
        n205 = Enqueue Element(queue=w485, element="Anatomia", error in (no error)=w479) -> (queue out=w483:refnum<queue>, error out=w478:errorcluster)  [unwired: 1 in, 1 out]
      }
      event Mouse Down? {
        n206 = event-data() -> ("Button"=w494:u16)  [unwired: 1 in, 7 out]
        n207 = Equal?(x=w494, y=u16 2) -> (x = y?=w492:bool)
        n208 = case shown="True" w492 {
          selector: w492 -> [w495 w496]
          tunnel: [w495 w496] -> w491
          frame False {
          }
          frame True {
          }
        }
        n209 = event-data("Discard?"=w491) -> ()  [unwired: 1 in, 1 out]
      }
      event "Kinect 1": Value Change {
        n210 = event-data() -> ()  [unwired: 1 in, 6 out]
        n211 = local read "Kinect 1"() -> (w504:bool)
        n212 = case shown="True" w504 {
          tunnel: w503 -> [w506 w511]
          tunnel: [w506 w510] -> w502
          tunnel: w501 -> [w505 w508]
          tunnel: [w505 w507] -> w500
          frame False {
          }
          frame True {
            n213 = Enqueue Element(queue=w511, element="ElevaçãoKinect1", error in (no error)=w508) -> (queue out=w510:refnum<queue>, error out=w507:errorcluster)  [unwired: 1 in, 1 out]
          }
        }
      }
      event "RGB": Value Change {
        n214 = event-data() -> ()  [unwired: 1 in, 6 out]
        n215 = Enqueue Element(queue=w519, element="CameraRGB", error in (no error)=w516) -> (queue out=w518:refnum<queue>, error out=w517:errorcluster)  [unwired: 1 in, 1 out]
      }
      event "Kinect 1": Value Change {
        w521 = T2."Enabled" ("Disabled")
        n216 = event-data() -> ()  [unwired: 1 in, 6 out]
        n217 = property on="RGB" class="Bool"("DisabledEnum"=w521) -> ()  [unwired: 2 in, 2 out]
        n218 = Enqueue Element(queue=w528, element="Ativar Kinect 1", error in (no error)=w526) -> (queue out=w527:refnum<queue>, error out=w525:errorcluster)  [unwired: 1 in, 1 out]
        n219 = property on="kinect" class="CmbBox"("DisabledEnum"=w521) -> ()  [unwired: 2 in, 2 out]
      }
      event "Menus": Value Change {
        n220 = event-data() -> ()  [unwired: 1 in, 6 out]
        n221 = Enqueue Element(queue=w535, element="Menus", error in (no error)=w536) -> (queue out=w534:refnum<queue>, error out=w533:errorcluster)  [unwired: 1 in, 1 out]
      }
    }
  }
  n222 = flat-sequence {
    tunnel: w10 -> [w538]
    tunnel: w5 -> [w537]
    frame #0 {
      n223 = call-poly <vilib>:"Kinect Close.vi"("Kinect References in"=w538, "error in"=w537) -> ()  [unwired: 13 in, 1 out]
    }
  }
